vi "math_ua_cplx.vi"(0 "x":cdb[](array[numeric]) format="%0.2f") -> (1 "mean(x)":cdb format="%0.2f", 2 "ua(x)":cdb format="%0.2f", 3 "ua(x) [ppm]":cdb format="%0.2f", 4 "std(x)":cdb format="%0.2f")   [LabVIEW 2020, in "varilib.lvlib"]
doc: "Calculates type A uncertainty for complex number."
uses:
  varilib.lvlib
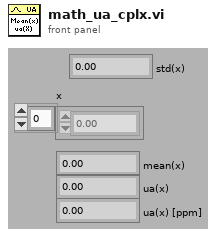
[diagram p1: front panel]
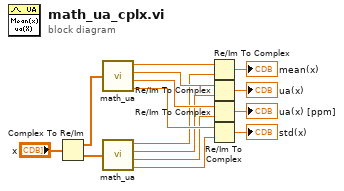
[diagram p0: block diagram]
diagram:
  n1 = Complex To Re/Im(x + iy="x") -> (x=w14:dbl[], y=w12:dbl[])
  n2 = call "math_ua.vi"("x"=w14) -> ("mean(x)"=w13:dbl, "ua(x)"=w11:dbl, "ua(x) [ppm]"=w10:dbl, "std(x)"=w9:dbl)
  n3 = call "math_ua.vi"("x"=w12) -> ("mean(x)"=w8:dbl, "ua(x)"=w7:dbl, "ua(x) [ppm]"=w6:dbl, "std(x)"=w5:dbl)
  n4 = Re/Im To Complex(1:w8, 2:w13) -> (0:→"mean(x)":cdb)
  n5 = Re/Im To Complex(1:w7, 2:w11) -> (0:→"ua(x)":cdb)
  n6 = Re/Im To Complex(1:w6, 2:w10) -> (0:→"ua(x) [ppm]":cdb)
  n7 = Re/Im To Complex(1:w5, 2:w9) -> (0:→"std(x)":cdb)
